vi "Actor Core.vi"(8 "error in":errorcluster, 11 "Select Report File Dialog in":refnum<class "Display Settings Dialog.lvclass">) -> (0 "error out":errorcluster, 3 "Actor out":refnum<class "Actor.lvclass">)   [LabVIEW 2014, in "Display Settings Dialog.lvlib" / "Display Settings Dialog.lvclass"]
doc: "(<B>Filename</B>: Actor Framework.lvlib:Actor.lvclass:Actor Core.vi)\n\nReceives messages to the actor, reacts to them, and initiates any error handling that may shut the actor down.\n\nDescendant classes may override this VI to append parallel tasks for the actor to complete while it handles messages. Overrides use the Call Parent Method node."
uses:
  Display Settings Dialog.lvclass
  <vilib>/ActorFramework/Actor/Actor.lvclass
  HIJ Vision Display/HIJ Vision Display/DisplaySettings.ctl
  <vilib>/ActorFramework/Actor/Actor.lvclass/Actor.ctl
  <vilib>/ActorFramework/Message Enqueuer/Message Enqueuer.lvclass/Message Enqueuer.ctl
  Display Settings Dialog.lvclass/Display Settings Dialog.ctl
  Display Settings Dialog Messages/Write Display settings Msg/Write Display settings Msg.lvclass/Write Display settings Msg.ctl
  HIJ Vision Display/HIJ Vision Display Messages/New Dispay Settings Msg/New Dispay Settings Msg.lvclass/New Dispay Settings Msg.ctl
  <vilib>/ActorFramework/Message Enqueuer/Init from Existing Queue.vi
  <vilib>/ActorFramework/Message Enqueuer/Enqueue.vi
  <vilib>/ActorFramework/Message Priority Queue/Priority Enqueue.vi
  Shared Code/Viewable Actor/ViewableActor/ViewableActor.lvclass
  <vilib>/ActorFramework/Message Enqueuer/Message Enqueuer.lvclass
  Display Settings Dialog Messages/Write Display settings Msg/Write Display settings Msg.lvclass
  HIJ Vision Display/HIJ Vision Display Messages/New Dispay Settings Msg/New Dispay Settings Msg.lvclass
  <vilib>/ActorFramework/Stop Msg/Stop Msg.lvclass
  HIJ Vision Display/HIJ Vision Display/HIJ Vision Display.lvclass
panel:
  in  "Display settings":T1={"Min. Thresh."=0.0, "X"=0.0, "Y"=0.0, "ShowLineout"=FALSE, "ScaleParts"=10, "ShowLegende"=FALSE, "Target Cross"=FALSE, "Centroid Cross"=FALSE, "Target color"=16777226, "Centroid color"=16711680, "calibr. µm/px"=0.0}
  in  "Stop Signal":bool
  in  "Stop":bool
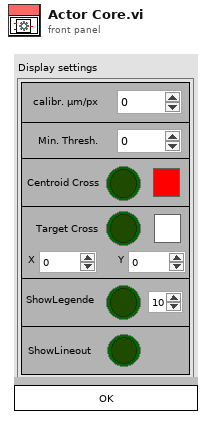
[diagram p1: front panel]
types:
  T1 = typedef "HIJ Vision Display.lvlib/HIJ Vision Display.lvclass/DisplaySettings.ctl" = cluster{"Min. Thresh.":sgl, "X":dbl, "Y":dbl, "ShowLineout":bool, "ScaleParts":i32, "ShowLegende":bool, "Target Cross":bool, "Centroid Cross":bool, "Target color":u32, "Centroid color":u32, "calibr. µm/px":sgl[unit]}
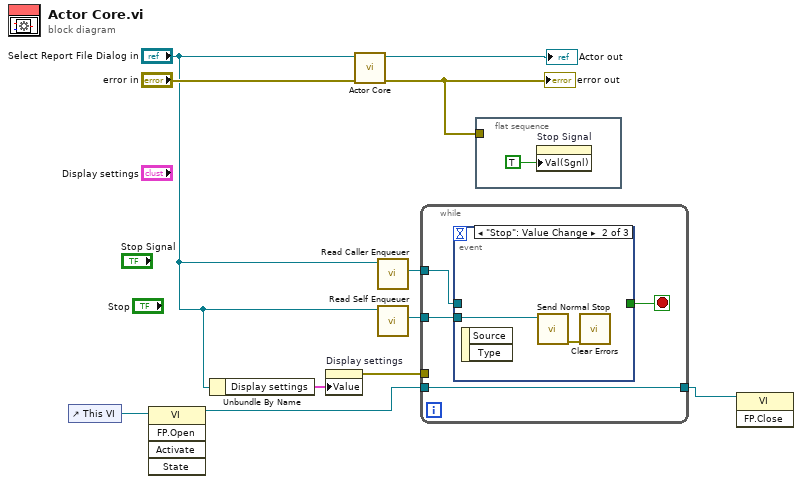
[diagram p0: block diagram]
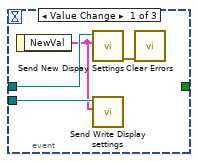
[diagram p2: hidden frame]
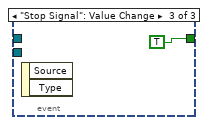
[diagram p3: hidden frame]
diagram:
  n1 = control-ref of="This VI"() -> (w7:refnum<vi>)
  n2 = invoke class="VI" method="FP.Open"(reference=w7) -> (reference out=w6:refnum<vi>)  [unwired: 4 in, 4 out]
  n3 = Unbundle By Name("Select Report File Dialog in") -> ("Display settings"=w2:T1)
  n4 = property on="Display settings" class="Clust (strict)"("Value"=w2) -> (error out=w1:errorcluster)  [unwired: 2 in, 1 out]
  n5 = call-parent "Actor Core.vi"("error in"="error in", "Actor in"="Select Report File Dialog in") -> ("error out"=w9:errorcluster, "Actor out"=→"Actor out":refnum<class "Actor.lvclass">)  [unwired: 8 in]
  "error out" <- w9
  n6 = call <vilib>:"Read Caller Enqueuer.vi"("Actor"="Select Report File Dialog in") -> ("Caller Enqueuer"=w4:refnum<class "Message Enqueuer.lvclass">)  [unwired: 10 in]
  n7 = call <vilib>:"Read Self Enqueuer.vi"("Actor"="Select Report File Dialog in") -> ("Self Enqueuer"=w8:refnum<class "Message Enqueuer.lvclass">)  [unwired: 10 in]
  n8 = while {
    tunnel: w8 -> [w15]
    tunnel: w6 -> [w13]
    tunnel: [w13] -> w5
    tunnel: w4 -> [w12]
    tunnel: w1 -> [_]
    stop <- w14 stop-if-true
    n9 = event shown="[1] \"Stop\": Value Change" {
      selector: _ -> [_ _ _]
      dyn-events: _ -> [_ _ _]
      timeout: _ -> [_ _ _]
      tunnel: w15 -> [w19 w21 _]
      tunnel: [_ _ TRUE] -> w14
      tunnel: w12 -> [w18 _ _]
      event Value Change {
        n10 = event-data() -> ("NewVal"=w17:T1)  [unwired: 1 in]
        n11 = call "Send New Dispay Settings.vi"("Display settings"=w17, "Message Enqueuer"=w18) -> ("error out"=w16:errorcluster)  [unwired: 8 in, 1 out]
        n12 = call "Send Write Display settings.vi"("Display settings"=w17, "Message Enqueuer"=w19) -> ()  [unwired: 8 in, 2 out]
        n13 = call <vilib>:"Clear Errors.vi"("error in (no error)"=w16) -> ()  [unwired: 5 in, 2 out]
      }
      event "Stop": Value Change {
        n14 = event-data() -> ()  [unwired: 1 in, 2 out]
        n15 = call <vilib>:"Send Normal Stop.vi"("Message Enqueuer"=w21) -> ("error out"=w20:errorcluster)  [unwired: 10 in]
        n16 = call <vilib>:"Clear Errors.vi"("error in (no error)"=w20) -> ()  [unwired: 5 in, 2 out]
      }
      event "Stop Signal": Value Change {
        n17 = event-data() -> ()  [unwired: 1 in, 2 out]
      }
    }
  }
  n18 = flat-sequence {
    tunnel: w9 -> [_]
    frame #0 {
      n19 = property on="Stop Signal" class="Bool (strict)"("Val(Sgnl)"=TRUE ("Value (Signaling)")) -> ()  [unwired: 2 in, 2 out]
    }
  }
  n20 = invoke class="VI" method="FP.Close"(reference=w5) -> ()  [unwired: 2 in, 3 out]
